vi "SampledValues.vi"() -> ()   [LabVIEW 2011]
uses:
  <vilib>/DAQmx/create/channels.llb/DAQmx Create Channel (AI-Voltage-Basic).vi
  <vilib>/DAQmx/configure/timing.llb/DAQmx Timing (Sample Clock).vi
  <vilib>/DAQmx/read.llb/DAQmx Read (Analog DBL 1Chan 1Samp).vi
panel:
  out "data":dbl format="%0.2f"
  in  "rate":dbl=1000.0 format="%0.2f"
  in  "physical channels":tag
  in  "minimum value":dbl=-5.0 format="%0.2f"
  in  "maximum value":dbl=5.0 format="%0.2f"
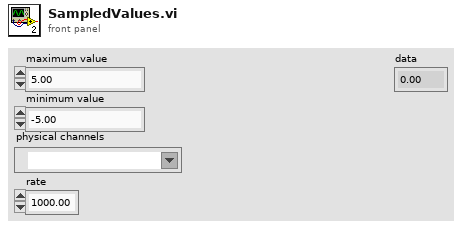
[diagram p1: front panel]
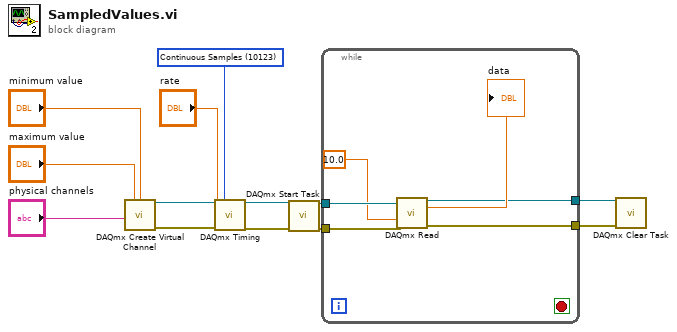
[diagram p0: block diagram]
diagram:
  w3 = 10123 items=["Finite Samples"=10178, "Continuous Samples"=10123, "Hardware Timed Single Point"=12522] ("sample mode")
  n1 = call-poly <vilib>:"DAQmx Create Virtual Channel.vi"("maximum value"="maximum value", "minimum value"="minimum value", "physical channels"="physical channels") -> ("task out"=w6:refnum<k21>, "error out"=w13:errorcluster)  [unwired: 11 in]
  n2 = call-poly <vilib>:"DAQmx Timing.vi"("task/channels in"=w6, "sample mode"=w3, "rate"="rate", "error in"=w13) -> ("task out"=w5:refnum<k21>, "error out"=w12:errorcluster)  [unwired: 10 in]
  n3 = call <vilib>:"DAQmx Start Task.vi"("task/channels in"=w5, "error in"=w12) -> ("task out"=w4:refnum<k21>, "error out"=w11:errorcluster)  [unwired: 12 in]
  n4 = while {
    tunnel: w11 -> [w19]
    tunnel: w4 -> [w18]
    tunnel: [w15] -> w2
    tunnel: [w14] -> w1
    stop <- _ stop-if-true
    n5 = call-poly <vilib>:"DAQmx Read.vi"("task/channels in"=w18, "timeout"=10.0, "error in"=w19) -> ("task out"=w15:refnum<k21>, "data"=→"data":dbl, "error out"=w14:errorcluster)  [unwired: 10 in]
  }
  n6 = call <vilib>:"DAQmx Clear Task.vi"("task in"=w2, "error in"=w1) -> ()  [unwired: 13 in, 1 out]
